vi "DSF.Engine.Transfer.Initialize.vi"(8 "error in (no error)":errorcluster, 10 "Transfer Configuration":refnum<class "DSF.Shared.Configuration.Transfer.lvclass">, 11 "Transfer type":refnum<class "DSF.Engine.Transfer.lvclass">) -> (0 "error out":errorcluster, 3 "Transfer out":refnum<class "DSF.Engine.Transfer.lvclass">)   [LabVIEW 2016, in "DSF.Engine.lvlib" / "DSF.Engine.Transfer.lvclass"]
uses:
  DSF.Engine.Transfer.lvclass
  Shared/Classes/Transfer/DSF.Shared.Configuration.Transfer.lvclass
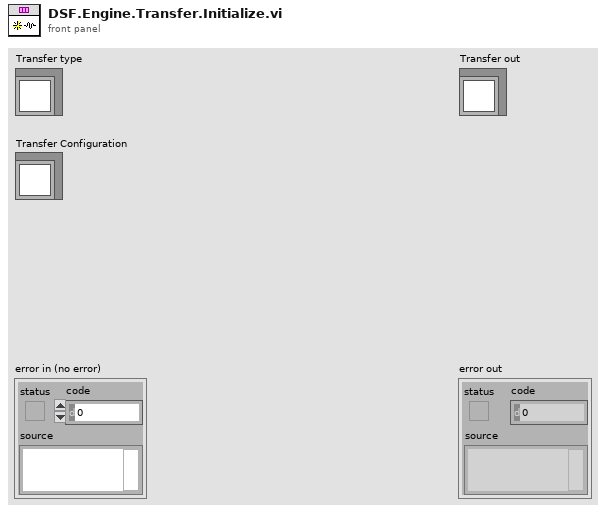
[diagram p1: front panel]
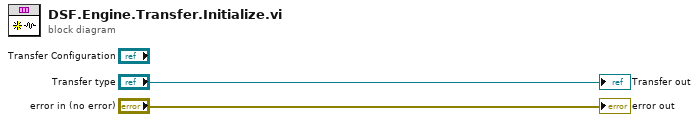
[diagram p0: block diagram]
diagram:
  "error out" <- "error in (no error)"
  "Transfer out" <- "Transfer type"
